vi "Configure Channel Output Level.vi"(0 "DG645 in":refnum<class "DG645.lvclass">, 1 "Rising Channel":T1, 2 "Falling Channel":T1, 3 "Amplitude":dbl, 4 "Offset":dbl, 5 "error in (no error)":errorcluster, 7 "Polarity (Positive:T)":bool=TRUE) -> (14 "DG645 out":refnum<class "DG645.lvclass">, 19 "error out":errorcluster)   [LabVIEW 2018, in "DG645.lvlib" / "DG645.lvclass"]
uses:
  DG645.lvclass
  PPLs/Digital Delay Generator/Parent/Digital Delay Generator.lvlibp/Custom Controls/Channel.ctl
  DG645.lvclass/DG645.ctl
  <instrlib>/Stanford Research DG645/Stanford Research DG645.lvlib
  PPLs/Digital Delay Generator/Parent/Digital Delay Generator.lvlibp/Digital Delay Generator.lvclass
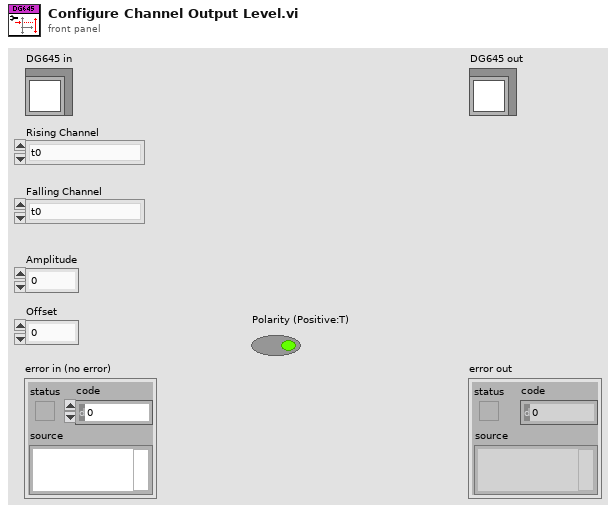
[diagram p1: front panel]
types:
  T1 = typedef "Digital Delay Generator.lvlibp/Digital Delay Generator.lvclass/Channel.ctl" = enum16{"t0", "A", "B", "C", "D", "E", "F", "G", "H"}
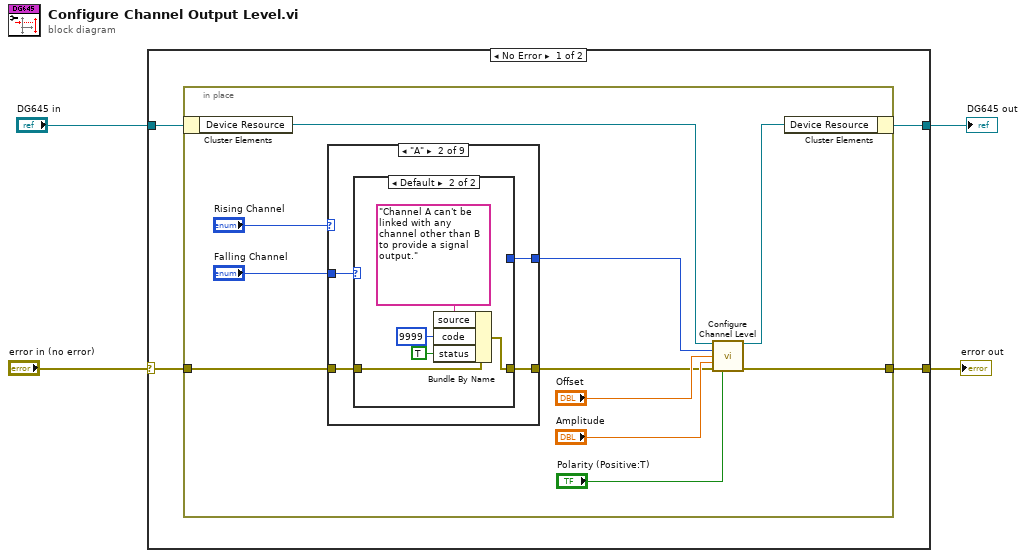
[diagram p0: block diagram]
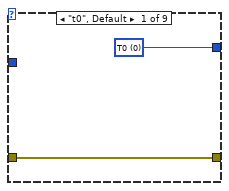
[diagram p2: hidden frame]
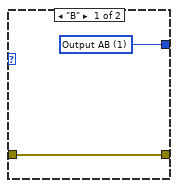
[diagram p3: hidden frame]
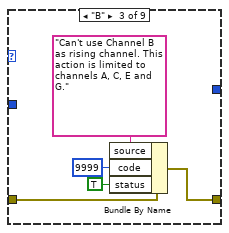
[diagram p4: hidden frame]
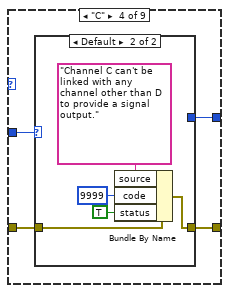
[diagram p5: hidden frame]
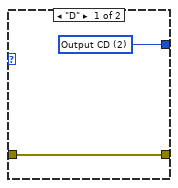
[diagram p6: hidden frame]
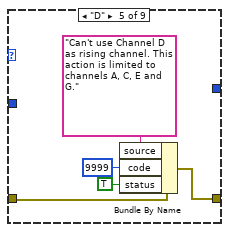
[diagram p7: hidden frame]
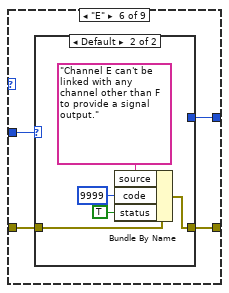
[diagram p8: hidden frame]
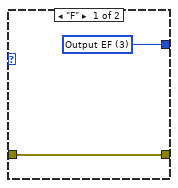
[diagram p9: hidden frame]
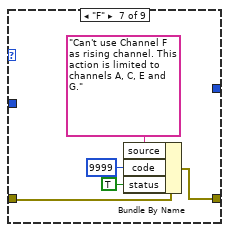
[diagram p10: hidden frame]
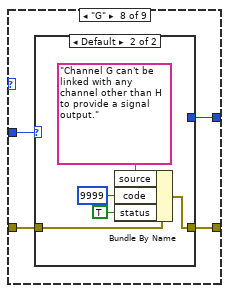
[diagram p11: hidden frame]
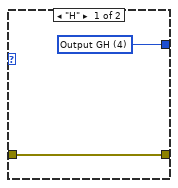
[diagram p12: hidden frame]
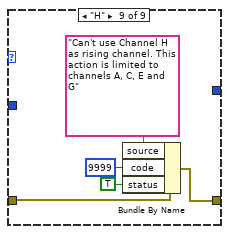
[diagram p13: hidden frame]
diagram:
  n1 = case shown="No Error" "error in (no error)" {
    selector: "error in (no error)" -> [w7 w87]
    tunnel: [w6 w87] -> w3
    tunnel: "DG645 in" -> [w8 w86]
    tunnel: [w5 w86] -> w1
    frame No Error {
      n2 = in-place {
        in-place-border: w7 -> [w13]
        in-place-border: [w19] -> w6
        n3 = in-place-cluster #1(w8) -> ("Device Resource"=w18:refnum<visa-resource-name>)
        n4 = case shown="\"A\"" "Rising Channel" {
          tunnel: [w21 w24 _ w40 _ w56 _ w72 _] -> w14
          tunnel: "Falling Channel" -> [_ w25 _ w41 _ w57 _ w73 _]
          tunnel: w13 -> [w20 w23 w34 w39 w50 w55 w66 w71 w82]
          tunnel: [w20 w22 w33 w38 w49 w54 w65 w70 w81] -> w12
          frame "t0", Default {
            w21 = u16 0 items=["T0", "Output AB", "Output CD", "Output EF", "Output GH"] ("Output Channel (0:T0)")
          }
          frame "A" {
            n5 = case shown="Default" w25 {
              tunnel: [w27 _] -> w24
              tunnel: w23 -> [w26 w32]
              tunnel: [w26 w31] -> w22
              frame "B" {
                w27 = u16 1 items=["T0", "Output AB", "Output CD", "Output EF", "Output GH"] ("Output Channel (0:T0)")
              }
              frame Default {
                n6 = Bundle By Name(cluster=w32, "source"="Channel A can't be linked with any channel other than B to provide a signal output.", "code"=9999, "status"=TRUE) -> (w31:errorcluster)
              }
            }
          }
          frame "B" {
            n7 = Bundle By Name(cluster=w34, "source"="Can't use Channel B as rising channel. This action is limited to channels A, C, E and G.", "code"=9999, "status"=TRUE) -> (w33:errorcluster)
          }
          frame "C" {
            n8 = case shown="Default" w41 {
              tunnel: [w43 _] -> w40
              tunnel: w39 -> [w42 w48]
              tunnel: [w42 w47] -> w38
              frame "D" {
                w43 = u16 2 items=["T0", "Output AB", "Output CD", "Output EF", "Output GH"] ("Output Channel (0:T0)")
              }
              frame Default {
                n9 = Bundle By Name(cluster=w48, "source"="Channel C can't be linked with any channel other than D to provide a signal output.", "code"=9999, "status"=TRUE) -> (w47:errorcluster)
              }
            }
          }
          frame "D" {
            n10 = Bundle By Name(cluster=w50, "source"="Can't use Channel D as rising channel. This action is limited to channels A, C, E and G.", "code"=9999, "status"=TRUE) -> (w49:errorcluster)
          }
          frame "E" {
            n11 = case shown="Default" w57 {
              tunnel: [w59 _] -> w56
              tunnel: w55 -> [w58 w64]
              tunnel: [w58 w63] -> w54
              frame "F" {
                w59 = u16 3 items=["T0", "Output AB", "Output CD", "Output EF", "Output GH"] ("Output Channel (0:T0)")
              }
              frame Default {
                n12 = Bundle By Name(cluster=w64, "source"="Channel E can't be linked with any channel other than F to provide a signal output.", "code"=9999, "status"=TRUE) -> (w63:errorcluster)
              }
            }
          }
          frame "F" {
            n13 = Bundle By Name(cluster=w66, "source"="Can't use Channel F as rising channel. This action is limited to channels A, C, E and G.", "code"=9999, "status"=TRUE) -> (w65:errorcluster)
          }
          frame "G" {
            n14 = case shown="Default" w73 {
              tunnel: [w75 _] -> w72
              tunnel: w71 -> [w74 w80]
              tunnel: [w74 w79] -> w70
              frame "H" {
                w75 = u16 4 items=["T0", "Output AB", "Output CD", "Output EF", "Output GH"] ("Output Channel (0:T0)")
              }
              frame Default {
                n15 = Bundle By Name(cluster=w80, "source"="Channel G can't be linked with any channel other than H to provide a signal output.", "code"=9999, "status"=TRUE) -> (w79:errorcluster)
              }
            }
          }
          frame "H" {
            n16 = Bundle By Name(cluster=w82, "source"="Can't use Channel H as rising channel. This action is limited to channels A, C, E and G", "code"=9999, "status"=TRUE) -> (w81:errorcluster)
          }
        }
        n17 = call <instrlib>:"Configure Channel Level.vi"("VISA resource name"=w18, "Positive Level Polarity (True)"="Polarity (Positive:T)", "Output Channel (0:T0)"=w14, "Level Offset (0 V)"="Offset", "Level Amplitude (2.5 V)"="Amplitude", "error in (no error)"=w12) -> ("VISA resource name out"=w17:refnum<visa-resource-name>, "error out"=w19:errorcluster)  [unwired: 8 in]
        n18 = in-place-cluster #1("Device Resource"=w17) -> (w5:refnum<class "DG645.lvclass">)
      }
    }
    frame Error {
    }
  }
  "error out" <- w3
  "DG645 out" <- w1
